vi "Parse Tree Labels.vi"(7 "Rx? (T:True, F: False (Tx))":bool, 8 "error out":errorcluster, 9 "Specified Channel Ref List":T1[](array[typedef]) format="%.0x", 10 "Label Refs":T1[](array[typedef]) format="%.0x", 11 "Custom Device Ref":T1 format="%.0x") -> (0 "error out":errorcluster, 3 "Label data":T2[](array[typedef]) {"Label Timestamp Channel Data Reference" format="%.0x"; "Label Disable/Trigger Channel Reference" format="%.0x"; "Word"."Param Setting"."Item Refs" format="%.0x"; "Word"."Param Setting"."Block Data Refs"."Data Reference" format="%.0x"; "Word"."Param Setting"."Num Bits" min=1 max=32; "Word"."Param Setting"."Start Bit" min=8 max=31; "Label" format="%.0o"})   [LabVIEW 2019, in "Ballard Arinc-429 System Explorer.lvlib"]
uses:
  Ballard Arinc-429 System Explorer.lvlib
  <vilib>/NI VeriStand/Custom Device API/Custom Device Item Ref.ctl
  Shared/Controls and Global/RT Label Settings.ctl
  Shared/Controls and Global/Label.ctl
  Shared/Controls and Global/transferPeriod.ctl
  Shared/Controls and Global/RT Word Settings.ctl
  Shared/Controls and Global/RT Param Setting.ctl
  Shared/Controls and Global/Start Bit.ctl
  Shared/Controls and Global/Number of Bits.ctl
  <vilib>/NI VeriStand/Custom Device API/Block Data Reference.ctl
  <vilib>/NI VeriStand/Custom Device API/Data Reference.ctl
  Shared/Controls and Global/TransferType.ctl
  <vilib>/NI VeriStand/Custom Device Tools/Custom Device Utility Library/Search Direction.ctl
  <vilib>/NI VeriStand/Custom Device API/Data Access Type.ctl
  Shared/Controls and Global/Global.vi
  <vilib>/NI VeriStand/Custom Device API/Get Item Property (U32).vi
  <vilib>/NI VeriStand/Custom Device API/Get Item Property (Boolean).vi
  <vilib>/NI VeriStand/Custom Device API/Get Item Property (String).vi
  <vilib>/NI VeriStand/Custom Device API/Get Item Property (U16).vi
  <vilib>/NI VeriStand/Custom Device Tools/Custom Device Utility Library/NI VeriStand - Search for Item by GUID.vi
  <vilib>/NI VeriStand/Custom Device Tools/Custom Device Utility Library/NI VeriStand - Search for All Items by GUID.vi
  <vilib>/NI VeriStand/Custom Device API/Get Item Property (I32).vi
  <vilib>/NI VeriStand/Custom Device API/Get Item Property (Double).vi
  <vilib>/NI VeriStand/Custom Device API/NI VeriStand - Get Channel Block Data References.vi
  <vilib>/NI VeriStand/Custom Device API/Custom Device API.lvlib
  Shared/Ballard Arinc-429 Shared.lvlib
  <vilib>/NI VeriStand/Custom Device Tools/Custom Device Utility Library/Custom Device Utility Library.lvlib
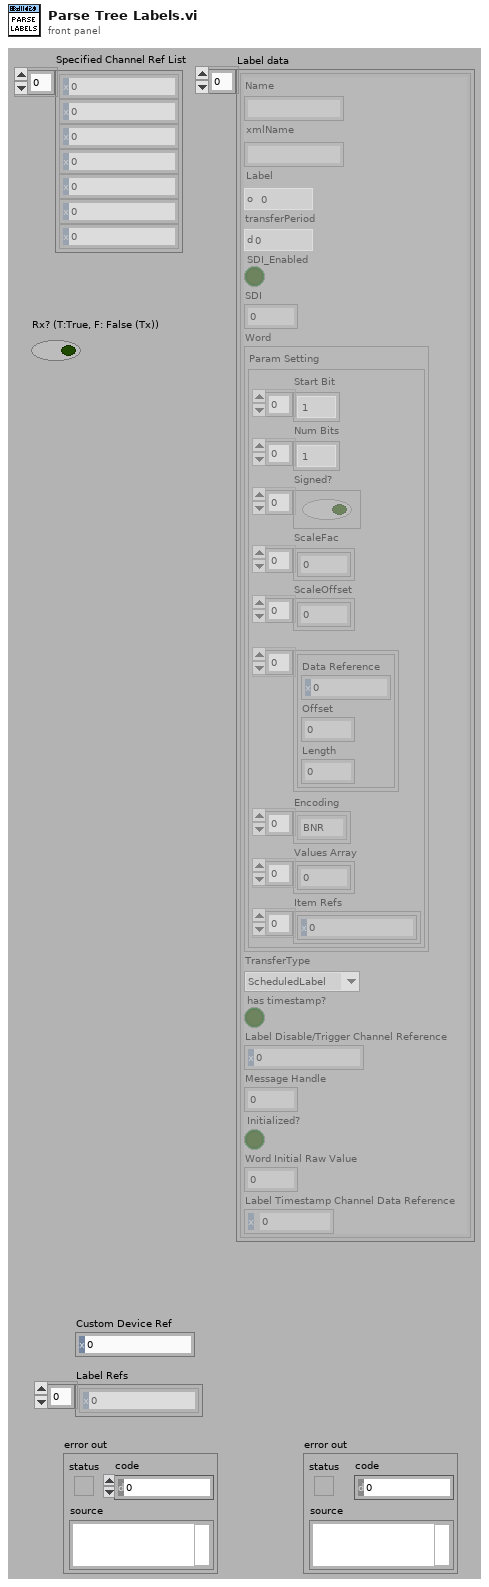
[diagram p1: front panel]
types:
  T1 = typedef "Custom Device API.lvlib/Custom Device Item Ref.ctl" = u64
  T2 = typedef "Ballard Arinc-429 Shared.lvlib/RT Label Settings.ctl" = cluster{"Name":string, "xmlName":string, "Label":T3, "transferPeriod":T4, "SDI_Enabled":bool, "SDI":u8, "Word":T5, "TransferType":T11, "has timestamp?":bool, "Label Disable/Trigger Channel Reference":T1, "Message Handle":u64, "Initialized?":bool, "Word Initial Raw Value":u32, "Label Timestamp Channel Data Reference":T10}
  T3 = typedef "Ballard Arinc-429 Shared.lvlib/Label.ctl" = u8
  T4 = typedef "Ballard Arinc-429 Shared.lvlib/transferPeriod.ctl" = u32
  T5 = typedef "Ballard Arinc-429 Shared.lvlib/RT Word Settings.ctl" = cluster{"Param Setting":T6}
  T6 = typedef "Ballard Arinc-429 Shared.lvlib/RT Param Setting.ctl" = cluster{"Start Bit":T7[], "Num Bits":T8[], "Signed?":bool[], "ScaleFac":dbl[], "ScaleOffset":dbl[], "Block Data Refs":T9[], "Encoding":enum16{"BNR", "BCD", "Discrete"}[], "Values Array":dbl[], "Item Refs":T1[]}
  T7 = typedef "Ballard Arinc-429 Shared.lvlib/Start Bit.ctl" = i32
  T8 = typedef "Ballard Arinc-429 Shared.lvlib/Number of Bits.ctl" = i32
  T9 = typedef "Custom Device API.lvlib/Block Data Reference.ctl" = cluster{"Data Reference":T10, "Offset":u64, "Length":u64}
  T10 = typedef "Custom Device API.lvlib/Data Reference.ctl" = i32
  T11 = typedef "Ballard Arinc-429 Shared.lvlib/TransferType.ctl" = enum16{"ScheduledLabel", "Acyclic", "Block", "Strobe"}
  T12 = typedef "Custom Device Utility Library.lvlib/Search Direction.ctl" = enum16{"Down", "Up"}
  T13 = typedef "Custom Device API.lvlib/Data Access Type.ctl" = enum16{"Read", "Write"}
  T14 = typedef "Custom Device API.lvlib/Custom Device Item Info.ctl" = cluster{"Name":string, "Is Channel":bool, "GUID":string, "Is Waveform":bool}
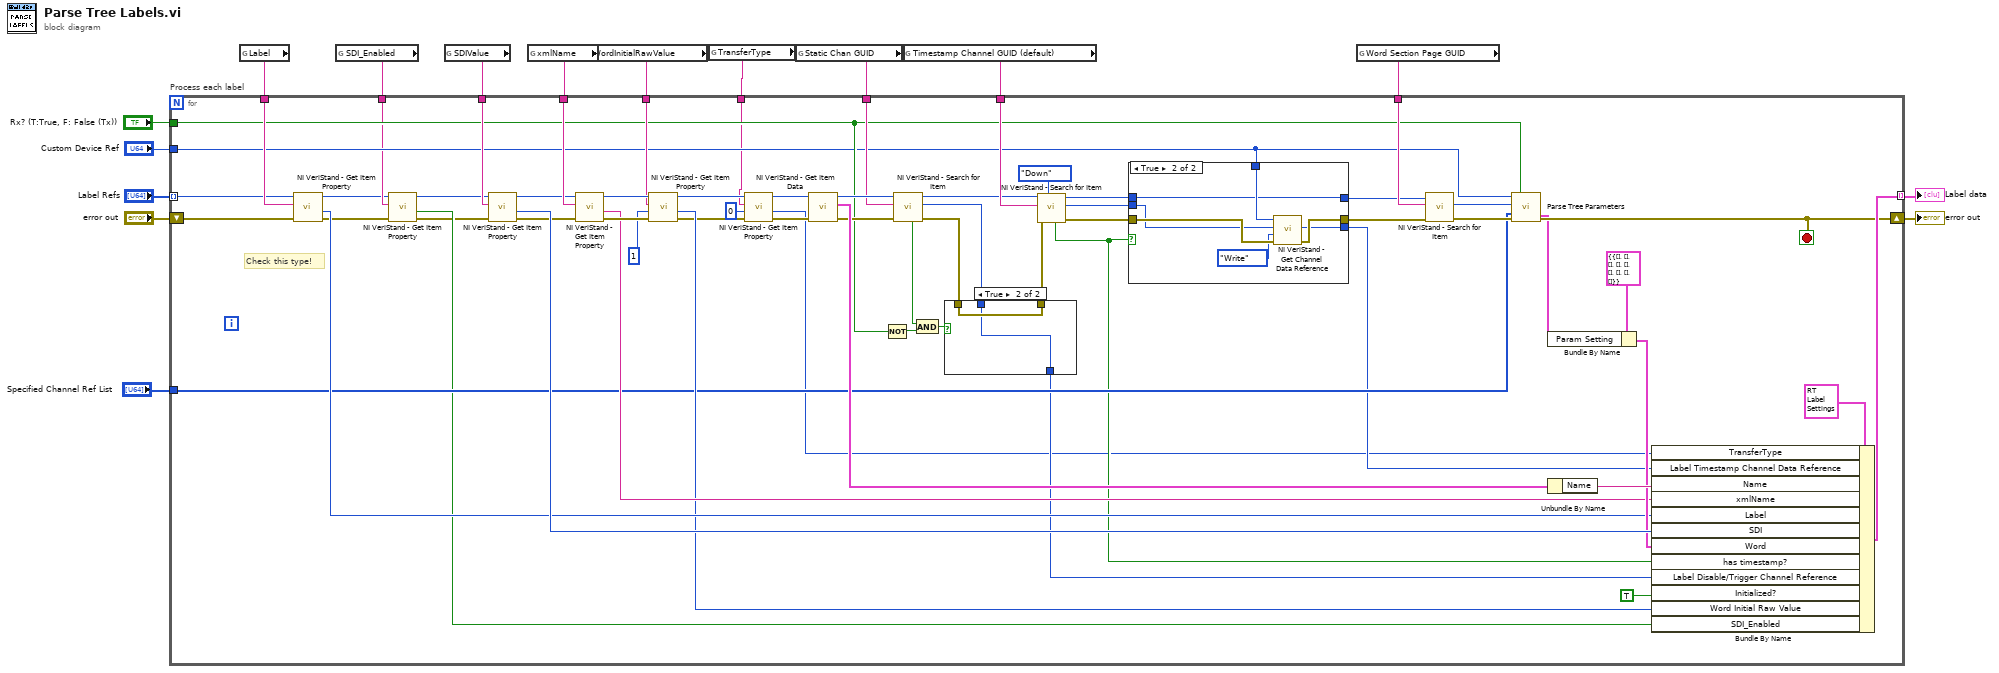
[diagram p0: block diagram]
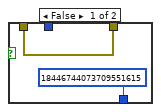
[diagram p3: hidden frame]
diagram:
  n1 = global read "Global.vi" "Label"() -> (w6:string)
  n2 = global read "Global.vi" "SDI_Enabled"() -> (w1:string)
  n3 = global read "Global.vi" "SDIValue"() -> (w12:string)
  n4 = global read "Global.vi" "xmlName"() -> (w11:string)
  n5 = global read "Global.vi" "WordInitialRawValue"() -> (w10:string)
  n6 = global read "Global.vi" "TransferType"() -> (w2:string)
  n7 = global read "Global.vi" "Static Chan GUID"() -> (w5:string)
  n8 = global read "Global.vi" "Timestamp Channel GUID (default)"() -> (w8:string)
  n9 = global read "Global.vi" "Word Section Page GUID"() -> (w9:string)
  n10 = for "Process each label" {
    tunnel: "Label Refs" -> [w61] mode=indexing
    shift-right: [w64] -> w13
    shift-left: "error out" -> [w63]
    tunnel: "Custom Device Ref" -> [w35]
    tunnel: w12 -> [w79]
    tunnel: w11 -> [w78]
    tunnel: w10 -> [w75]
    tunnel: w9 -> [w73]
    tunnel: w8 -> [w71]
    tunnel: [w68] -> w7 mode=indexing
    tunnel: w6 -> [w62]
    tunnel: w5 -> [w56]
    tunnel: "Specified Channel Ref List" -> [w44]
    tunnel: "Rx? (T:True, F: False (Tx))" -> [w43]
    tunnel: w2 -> [w25]
    tunnel: w1 -> [w22]
    stop <- w64 stop-if-true
    # "Check this type!"
    n11 = call-poly <vilib>:"NI VeriStand - Get Item Property.vi"("error in (no error)"=w63, "Property Name"=w62, "Item Ref in"=w61) -> ("error out"=w18:errorcluster, "Value"=w53:u32, "Item Ref out"=w20:T1)  [unwired: 5 in, 1 out]
    n12 = call-poly <vilib>:"NI VeriStand - Get Item Property.vi"("error in (no error)"=w18, "Property Name"=w22, "Item Ref in"=w20) -> ("error out"=w17:errorcluster, "Value"=w21:bool, "Item Ref out"=w19:T1)  [unwired: 5 in, 1 out]
    n13 = call-poly <vilib>:"NI VeriStand - Get Item Property.vi"("error in (no error)"=w17, "Property Name"=w79, "Item Ref in"=w19) -> ("error out"=w54:errorcluster, "Value"=w70:u32, "Item Ref out"=w55:T1)  [unwired: 5 in, 1 out]
    n14 = call-poly <vilib>:"NI VeriStand - Get Item Property.vi"("error in (no error)"=w54, "Property Name"=w78, "Item Ref in"=w55) -> ("error out"=w77:errorcluster, "Value"=w65:string, "Item Ref out"=w76:T1)  [unwired: 5 in, 1 out]
    n15 = call-poly <vilib>:"NI VeriStand - Get Item Property.vi"("error in (no error)"=w77, "Default Value"=u32 1, "Property Name"=w75, "Item Ref in"=w76) -> ("error out"=w28:errorcluster, "Value"=w45:u32, "Item Ref out"=w29:T1)  [unwired: 4 in, 1 out]
    n16 = call-poly <vilib>:"NI VeriStand - Get Item Property.vi"("error in (no error)"=w28, "Default Value"=u16 0, "Property Name"=w25, "Item Ref in"=w29) -> ("error out"=w27:errorcluster, "Value"=w23:u16, "Item Ref out"=w26:T1)  [unwired: 4 in, 1 out]
    n17 = call <vilib>:"NI VeriStand - Get Item Data.vi"("error in (no error)"=w27, "Item Ref in"=w26) -> ("error out"=w58:errorcluster, "Item Info"=w60:T14, "Item Ref out"=w57:T1)  [unwired: 6 in, 1 out]
    n18 = Not(x=w43) -> (.not. x?=w31:bool)
    n19 = call-poly <vilib>:"NI VeriStand - Search for Item.vi"("error in"=w58, "Item GUID"=w56, "Section Ref in"=w57) -> ("error out"=w52:errorcluster, "Item Ref"=w50:T1, "Section Ref out"=w49:T1, "Found"=w30:bool)  [unwired: 5 in]
    n20 = And(x=w30, y=w31) -> (x .and. y?=w32:bool)
    n21 = case shown="True" w32 {
      tunnel: w52 -> [w89 w92]
      tunnel: [w89 w92] -> w51
      tunnel: w50 -> [_ w91]
      tunnel: [T1 18446744073709551615 ("Item Ref") w91] -> w33
      frame False {
      }
      frame True {
      }
    }
    n22 = call-poly <vilib>:"NI VeriStand - Search for Item.vi"("Direction (Down)"=Search_Direction."Down", "error in"=w51, "Item GUID"=w71, "Section Ref in"=w49) -> ("error out"=w38:errorcluster, "Item Ref"=w42:T1, "Section Ref out"=w40:T1, "Found"=w41:bool)  [unwired: 4 in]
    n23 = case shown="True" w41 {
      tunnel: w42 -> [_ w85]
      tunnel: w40 -> [w81 w83]
      tunnel: [w81 w83] -> w39
      tunnel: w38 -> [w80 w88]
      tunnel: [w80 w86] -> w37
      tunnel: [_ w82] -> w36
      tunnel: w35 -> [_ w84]
      frame False {
      }
      frame True {
        n24 = call <vilib>:"NI VeriStand - Get Channel Data Reference.vi"("error in (no error)"=w88, "Access"=Data_Access_Type."Write", "Channel Ref in"=w85, "Device Ref in"=w84) -> ("error out"=w86:errorcluster, "Channel Data Reference"=w82:T10)  [unwired: 5 in, 1 out]
      }
    }
    n25 = call-poly <vilib>:"NI VeriStand - Search for Item.vi"("error in"=w37, "Item GUID"=w73, "Section Ref in"=w39) -> ("error out"=w74:errorcluster, "Item Ref"=w59:T1)  [unwired: 5 in, 2 out]
    n26 = call "Parse Tree Parameters.vi"("Custom Device Ref"=w35, "Rx? (T:True, F: False (Tx))"=w43, "Item Ref in"=w59, "Specified Channel Ref List"=w44, "error in"=w74) -> ("Parameter Driver Data"=w46:T6, "error out"=w64:errorcluster)  [unwired: 8 in, 1 out]
    n27 = Bundle By Name(cluster=T5 {"Param Setting"={"Start Bit"=[], "Num Bits"=[], "Signed?"=[], "ScaleFac"=[], "ScaleOffset"=[], "Block Data Refs"=[], "Encoding"=[], "Values Array"=[], "Item Refs"=[]}} ("Word"), "Param Setting"=w46) -> (w66:T5)
    n28 = Unbundle By Name(w60) -> ("Name"=w69:string)
    n29 = Bundle By Name(cluster=T2 {"Name"="", "xmlName"="", "Label"=0, "transferPeriod"=0, "SDI_Enabled"=FALSE, "SDI"=0, "Word"={"Param Setting"={"Start Bit"=[], "Num Bits"=[], "Signed?"=[], "ScaleFac"=[], "ScaleOffset"=[], "Block Data Refs"=[], "Encoding"=[], "Values Array"=[], "Item Refs"=[]}}, "TransferType"=enum."ScheduledLabel", "has timestamp?"=FALSE, "Label Disable/Trigger Channel Reference"=0, "Message Handle"=0, "Initialized?"=FALSE, "Word Initial Raw Value"=0, "Label Timestamp Channel Data Reference"=0} ("Label Settings"), "TransferType"=w23, "Label Timestamp Channel Data Reference"=w36, "Name"=w69, "xmlName"=w65, "Label"=w53, "SDI"=w70, "Word"=w66, "has timestamp?"=w41, "Label Disable/Trigger Channel Reference"=w33, "Initialized?"=TRUE, "Word Initial Raw Value"=w45, "SDI_Enabled"=w21) -> (w68:T2)
  }
  "Label data" <- w7
  "error out" <- w13
